vi "softwareTrigger_action.vi"(0 "HGF_BaslerDx":refnum<class "HGF_BaslerDx.lvclass">, 5 "error in (no error)":errorcluster) -> (14 "dup HGF_BaslerDx":refnum<class "HGF_BaslerDx.lvclass">, 19 "error out":errorcluster)   [LabVIEW 2014, in "HGF_IMAQ.lvlib" / "HGF_BaslerDx.lvclass"]
doc: "Generate a software trigger."
uses:
  HGF_BaslerDx.lvclass
  HGF_VisionTools/HGF_VisionTools.lvlib
  HGF_VisionTools/IMAQdx_setAttribute_Enum.vi
  HGF_ImaqDx/HGF_ImaqDx.lvclass
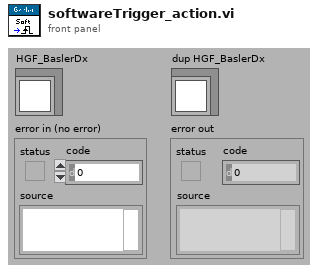
[diagram p1: front panel]
types:
  T1 = typedef "IMAQdx.ctl" = refnum<k21>
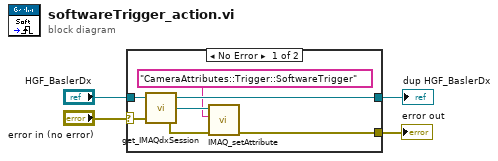
[diagram p0: block diagram]
diagram:
  n1 = case shown="No Error" "error in (no error)" {
    selector: "error in (no error)" -> [w9 w12]
    tunnel: "HGF_BaslerDx" -> [w10 w13]
    tunnel: [w7 w13] -> w2
    tunnel: [w5 w12] -> w1
    frame No Error {
      n2 = call "get_IMAQdxSession.vi"("error in (no error)"=w9, "HGF_ImaqDx in"=w10) -> ("error out"=w8:errorcluster, "IMAQdx Session"=w11:T1, "HGF_ImaqDx out"=w7:refnum<class "HGF_BaslerDx.lvclass">)  [unwired: 1 in]
      n3 = call-poly "IMAQ_setAttribute.vi"("error in (no error)"=w8, "Attribute Name"="CameraAttributes::Trigger::SoftwareTrigger", "IMAQdx Session"=w11) -> ("error out"=w5:errorcluster)  [unwired: 2 in, 2 out]
    }
    frame Error {
    }
  }
  "error out" <- w1
  "dup HGF_BaslerDx" <- w2
